vi "Multiply Array by Scalar.vi"(1 "1D Array":dbl[](array[numeric]), 4 "Scaling Factor":dbl) -> (15 "Scaled 1D Array":dbl[](array[numeric]))   [LabVIEW 2014]
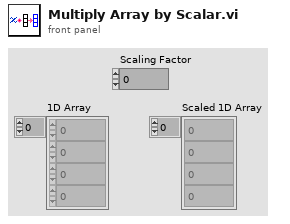
[diagram p1: front panel]
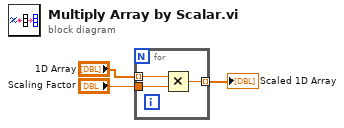
[diagram p0: block diagram]
diagram:
  n1 = for {
    tunnel: "1D Array" -> [w6] mode=indexing
    tunnel: "Scaling Factor" -> [w5]
    tunnel: [w4] -> w1 mode=indexing
    n2 = Multiply(x=w6, y=w5) -> (x*y=w4:dbl)
  }
  "Scaled 1D Array" <- w1
